vi "Finding Remote.vi"() -> (0 "Final":i32, 1 "Found??":bool, 2 "Current":i32)   [LabVIEW 2015]
uses:
  <vilib>/Utility/inputDevices.llb/joystickAcquire.vi
  <vilib>/Utility/inputDevices.llb/closeJoystick.vi
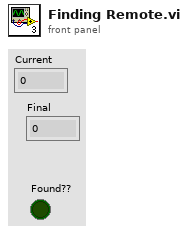
[diagram p1: front panel]
types:
  T1 = cluster{"button 1":bool, "button 2":bool, "button 3":bool, "button 4":bool, "button 5":bool, "button 6":bool, "button 7":bool, "button 8":bool, "button 9":bool, "button 10":bool, "button 11":bool, "button 12":bool, "button 13":bool, "button 14":bool, "button 15":bool, "button 16":bool, "button 17":bool, "button 18":bool, "button 19":bool, "button 20":bool, "button 21":bool, "button 22":bool, "button 23":bool, "button 24":bool, "button 25":bool, "button 26":bool, "button 27":bool, "button 28":bool, "button 29":bool, "button 30":bool, "button 31":bool, "button 32":bool}
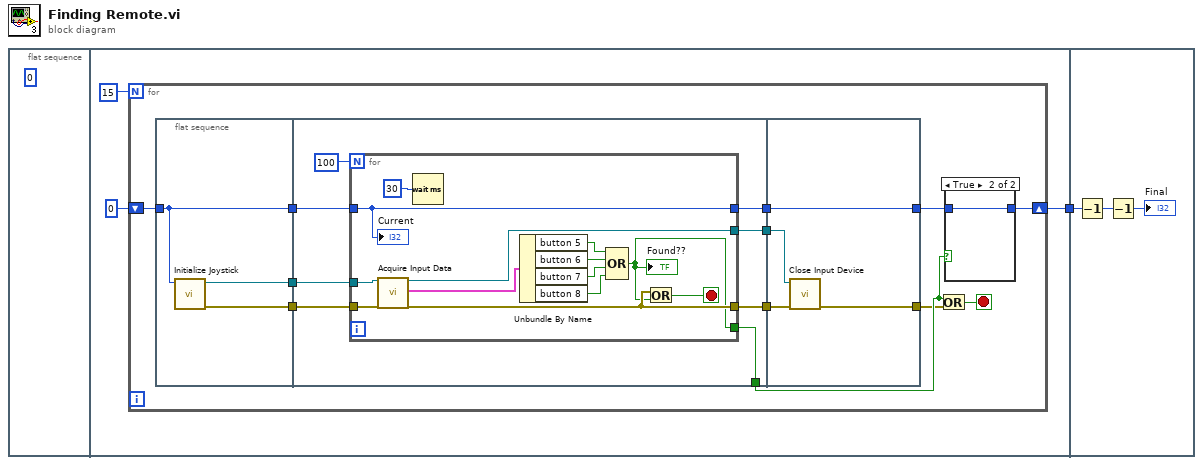
[diagram p0: block diagram]
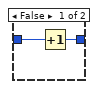
[diagram p2: hidden frame]
diagram:
  n1 = flat-sequence {
    tunnel: [w2] -> w1
    tunnel: w1 -> [w50]
    frame #0 {
      (unwired) 0 ("Actual Channel")
    }
    frame #1 {
      n2 = for {
        N: 15 -> [_]
        shift-right: [w13] -> w2
        shift-left: 0 -> [w14]
        stop <- w8 stop-if-true
        n3 = flat-sequence {
          tunnel: [w22] -> w16
          tunnel: [w20] -> w15
          tunnel: w14 -> [w21]
          tunnel: [w21] -> w12
          tunnel: w16 -> [w29]
          tunnel: w15 -> [w28]
          tunnel: w12 -> [w27]
          tunnel: [w23] -> w11
          tunnel: [w26] -> w10
          tunnel: [w25] -> w9
          tunnel: [w24] -> w6
          tunnel: [w47] -> w7
          tunnel: w11 -> [w47]
          tunnel: w10 -> [w46]
          tunnel: w9 -> [w45]
          tunnel: [w44] -> w5
          frame #0 {
            n4 = call <vilib>:"Initialize Joystick.vi"("device index"=w21) -> ("error out"=w20:errorcluster, "device ID"=w22:refnum<k1>)  [unwired: 9 in]
          }
          frame #1 {
            n5 = for {
              N: 100 -> [_]
              tunnel: w29 -> [w43]
              tunnel: w28 -> [w42]
              tunnel: w27 -> [w32]
              tunnel: [w32] -> w23
              tunnel: [w41] -> w26
              tunnel: [w35] -> w25
              tunnel: [w31] -> w24
              stop <- w34 stop-if-true
              n6 = call-poly <vilib>:"Acquire Input Data.vi"("device ID"=w43, "error in (no error)"=w42) -> ("device ID"=w41:refnum<k1>, "button info"=w40:T1, "error out"=w35:errorcluster)  [unwired: 13 in, 2 out]
              n7 = Wait (ms)(milliseconds to wait=u32 30) -> ()  [unwired: 1 out]
              n8 = Unbundle By Name(w40) -> ("button 5"=w39:bool, "button 6"=w38:bool, "button 7"=w37:bool, "button 8"=w36:bool)
              n9 = Compound Arithmetic op=OR(w39, w38, w37, w36) -> (w31:bool)
              "Found??" <- w31
              n10 = Or(x=w35, y=w31) -> (x .or. y?=w34:bool)
              "Current" <- w32
            }
          }
          frame #2 {
            n11 = call-poly <vilib>:"Close Input Device.vi"("error in (no error)"=w45, "device ID"=w46) -> ("error out"=w44:errorcluster)  [unwired: 8 in]
          }
        }
        n12 = Or(x=w6, y=w5) -> (x .or. y?=w8:bool)
        n13 = case shown="True" w6 {
          tunnel: [w18 w19] -> w13
          tunnel: w7 -> [w17 w19]
          frame False {
            n14 = Increment(x=w17) -> (x+1=w18:i32)
          }
          frame True {
          }
        }
      }
    }
    frame #2 {
      n15 = Decrement(x=w50) -> (x-1=w49:i32)
      n16 = Decrement(x=w49) -> (x-1=→"Final":i32)
    }
  }
